vi "MuxSwitchSingle.vi"(7 "MUX address":u32=1 min=1 max=12 step=1, 8 "error in (no error)":errorcluster, 9 "Channel":i32=1 min=1 max=12 step=1, 10 "Bank":i32=1 min=1 max=12 step=1, 11 "LXIPXISwitching in":refnum<class "LXIPXISwitching.lvclass">) -> (0 "error out":errorcluster, 2 "command string":string, 3 "LXIPXISwitching out":refnum<class "LXIPXISwitching.lvclass">)   [LabVIEW 2019, in "LXIPXISwitching.lvclass"]
uses:
  LXIPXISwitching.lvclass
  InstrumentSetup.vi
  InstrControl.lvclass
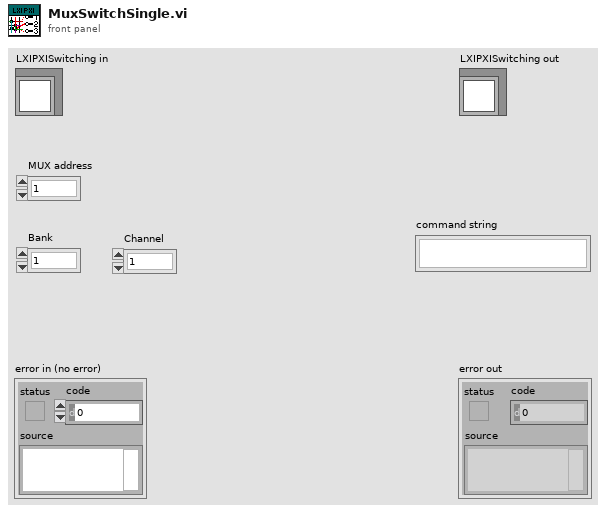
[diagram p1: front panel]
types:
  T1 = cluster{"MUX":string, "Matrix":string, "Breadboard":string, "LXIPXI Switching":refnum<class "LXIPXISwitching.lvclass">, "MUX PN":string, "Matrix  PN":string, "Breadboard PN":string, "MUX ID":string, "Matrix ID":string, "Breadboard ID":string, "LCR?":bool, "SMU?":bool}
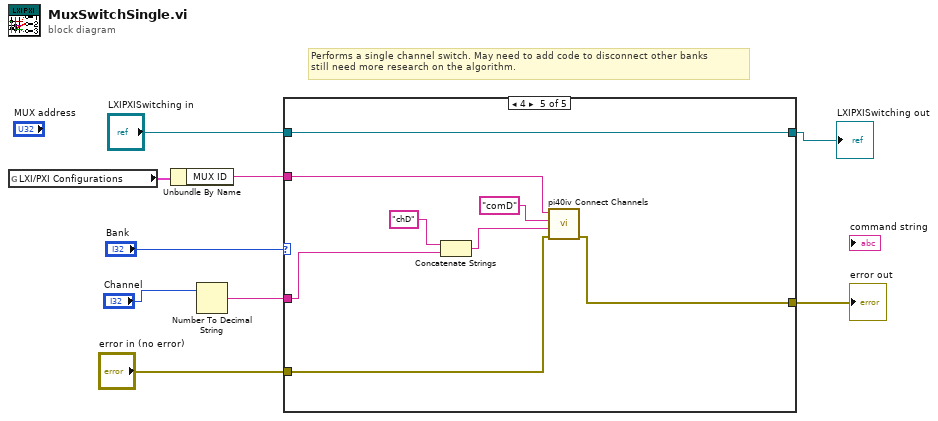
[diagram p0: block diagram]
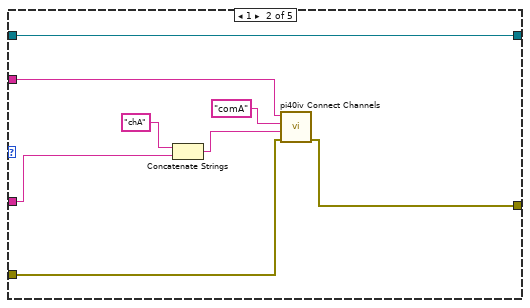
[diagram p3: hidden frame]
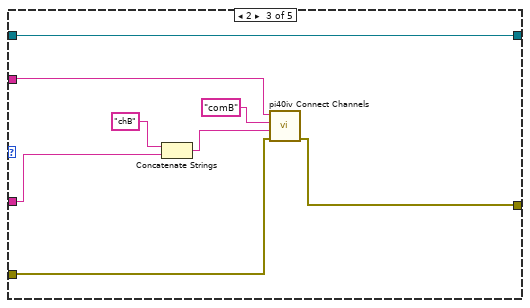
[diagram p4: hidden frame]
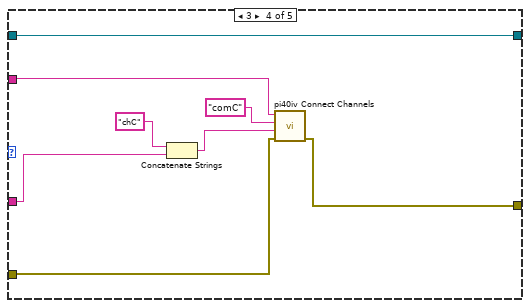
[diagram p5: hidden frame]
diagram:
  # "Performs a single channel switch. May need to add code to disconnect other banks\nstill need more research on the algorithm."
  n1 = global read "InstrumentSetup.vi" "LXI/PXI Configurations"() -> (w9:T1)
  n2 = Unbundle By Name(w9) -> ("MUX ID"=w8:string)
  n3 = Number To Decimal String(number="Channel") -> (decimal integer string=w3:string)  [unwired: 1 in]
  n4 = case shown="4" "Bank" {
    tunnel: w8 -> [_ w14 w23 w32 w43]
    tunnel: "error in (no error)" -> [w10 w16 w22 w30 w41]
    tunnel: [w10 w13 w24 w29 w40] -> w6
    tunnel: w3 -> [_ w15 w21 w31 w39]
    tunnel: "LXIPXISwitching in" -> [w11 w12 w20 w28 w36]
    tunnel: [w11 w12 w20 w28 w36] -> w1
    frame 0, Default {
    }
    frame 1 {
      n5 = Concatenate Strings("chA" ("string"), w15) -> (w17:string)
      n6 = call <instrlib>:"pi40iv Connect Channels.vi"("error in (no error)"=w16, "channel 2"=w17, "channel 1"="comA", "instrument handle"=w14) -> ("error out"=w13:errorcluster)  [unwired: 6 in, 1 out]
    }
    frame 2 {
      n7 = Concatenate Strings("chB" ("string"), w21) -> (w25:string)
      n8 = call <instrlib>:"pi40iv Connect Channels.vi"("error in (no error)"=w22, "channel 2"=w25, "channel 1"="comB", "instrument handle"=w23) -> ("error out"=w24:errorcluster)  [unwired: 6 in, 1 out]
    }
    frame 3 {
      n9 = Concatenate Strings("chC" ("string"), w31) -> (w33:string)
      n10 = call <instrlib>:"pi40iv Connect Channels.vi"("error in (no error)"=w30, "channel 2"=w33, "channel 1"="comC", "instrument handle"=w32) -> ("error out"=w29:errorcluster)  [unwired: 6 in, 1 out]
    }
    frame 4 {
      n11 = Concatenate Strings("chD" ("string"), w39) -> (w37:string)
      n12 = call <instrlib>:"pi40iv Connect Channels.vi"("error in (no error)"=w41, "channel 2"=w37, "channel 1"="comD", "instrument handle"=w43) -> ("error out"=w40:errorcluster)  [unwired: 6 in, 1 out]
    }
  }
  "error out" <- w6
  "LXIPXISwitching out" <- w1
